vi "Get Attribute Meta Data.vi"(7 "Unique ID":string, 8 "error in (no error)":errorcluster, 9 "Attribute Type":variant, 10 "Attribute Name":string, 11 "Test Executive Ref":refnum<data-value>) -> (0 "error out":errorcluster, 1 "Found?":bool, 2 "Meta Data":string, 3 "Test Executive Ref out":refnum<data-value>)   [LabVIEW 2020, in "Test Executive.lvlib" / "TestExecutive Ref.lvclass"]
uses:
  <vilib>/gpm_packages/@cs/test-executive/Source/Test Executive/TestExecutive Ref/TestExecutive Ref.lvclass
  <vilib>/gpm_packages/@cs/test-executive/Source/Test Executive/ITestExecutive/ITest Executive.lvclass
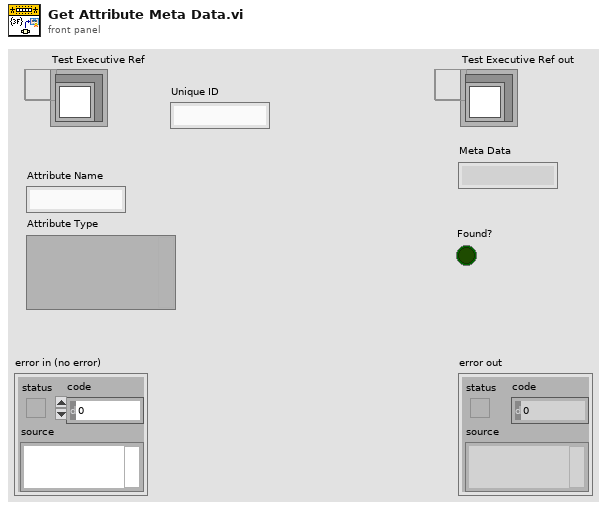
[diagram p1: front panel]
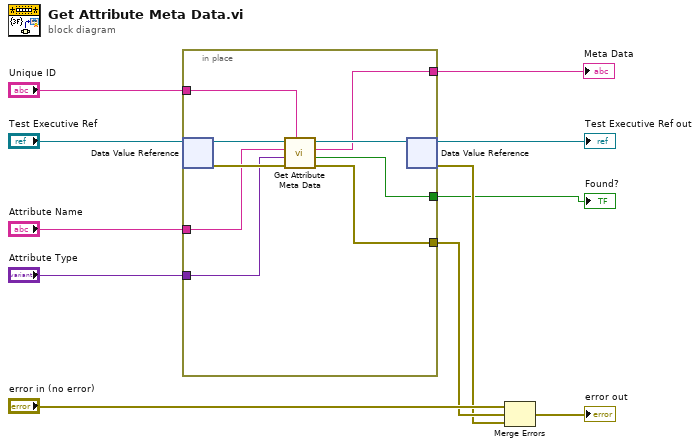
[diagram p0: block diagram]
diagram:
  n1 = in-place {
    in-place-border: "Unique ID" -> [w20]
    in-place-border: [w16] -> w7
    in-place-border: [w15] -> w4
    in-place-border: [w14] -> w3
    in-place-border: "Attribute Name" -> [w13]
    in-place-border: "Attribute Type" -> [w12]
    n2 = in-place-dvr #1("Test Executive Ref") -> (w19:refnum<class "ITest Executive.lvclass">, w17:errorcluster)
    n3 = call-dynamic "Get Attribute Meta Data.vi"("Unique ID"=w20, "error in (no error)"=w17, "Attribute Type"=w12, "Attribute Name"=w13, "ITest Executive in"=w19) -> ("error out"=w16:errorcluster, "Found?"=w14:bool, "Meta Data"=w15:string, "ITest Executive out"=w18:refnum<class "ITest Executive.lvclass">)  [unwired: 3 in]
    n4 = in-place-dvr #1(w18) -> (→"Test Executive Ref out":refnum<data-value>, w6:errorcluster)
  }
  "Meta Data" <- w4
  "Found?" <- w3
  n5 = Merge Errors("error in (no error)", w7, w6) -> (→"error out":errorcluster)
